vi "RFIDStart.vi"(0 "Device Info":T1={"Serial Number"=-1, "Channel"=0, "Port"=0}, 5 "AntennaState":bool=TRUE caption="Antenna Enabled", 11 "error in (no error)":errorcluster, 12 "Connection":u16(ring) items=["No Preference", "Remote", "Local"], 13 "Timeout (mSec)":i32=5000) -> (4 "Phidget ID":u64, 6 "Serial Number Return":i32, 10 "Attached?":bool, 15 "error out":errorcluster)   [LabVIEW 2012, in "Phidget RFID.lvlib"]
doc: "${RFID:StartHeader}"
uses:
  <instrlib>/Phidgets/Phidget RFID/Phidget RFID.lvlib
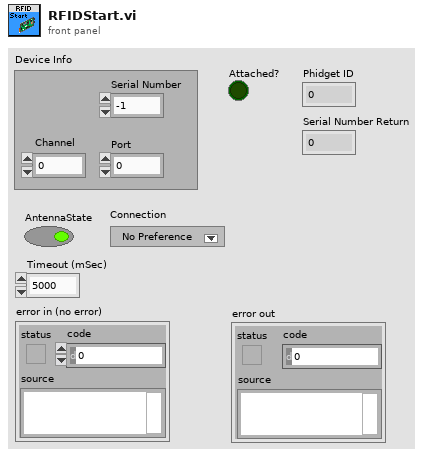
[diagram p1: front panel]
types:
  T1 = cluster{"Serial Number":i32, "Channel":i32, "Port":i32}
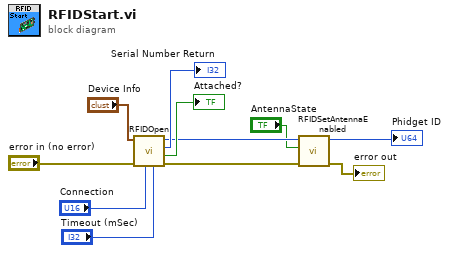
[diagram p0: block diagram]
diagram:
  n1 = call <instrlib>:"RFIDOpen.vi"("Timeout (mSec)"="Timeout (mSec)", "Network?"="Connection", "error in"="error in (no error)", "Device Info"="Device Info") -> ("error out"=w6:errorcluster, "Attached?"=→"Attached?":bool, "Serial Number Return"=→"Serial Number Return":i32, "Phidget ID"=w7:u64)  [unwired: 4 in]
  n2 = call <instrlib>:"RFIDSetAntennaEnabled.vi"("error in (no error)"=w6, "AntennaState"="AntennaState", "Device In"=w7) -> ("error out"=→"error out":errorcluster, "Device Out"=→"Phidget ID":u64)  [unwired: 6 in]
